vi "Config - Read.vi"(8 "error in (no error)":errorcluster, 11 "Filepath":path) -> (0 "error out":errorcluster, 3 "Config Array":T1 {"Balance" format="%9.2g"})   [LabVIEW 2017]
doc: "Provides READ all data from external config DB."
uses:
  Controls/Config Array.ctl
  Controls/Config Data.ctl
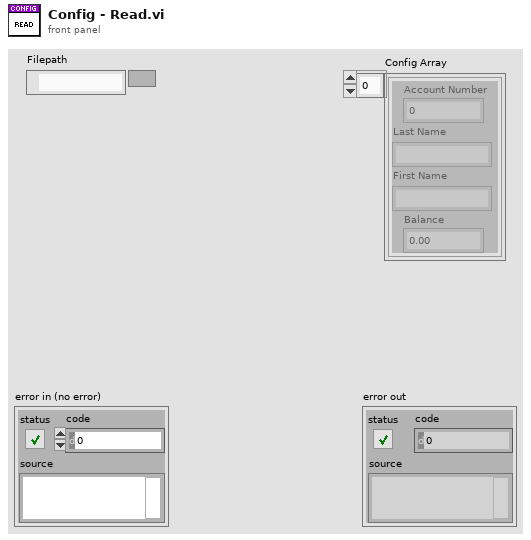
[diagram p1: front panel]
types:
  T1 = typedef "Config Array.ctl" = T2[]
  T2 = typedef "Config Data.ctl" = cluster{"Account Number":u32, "Last Name":string, "First Name":string, "Balance":dbl}
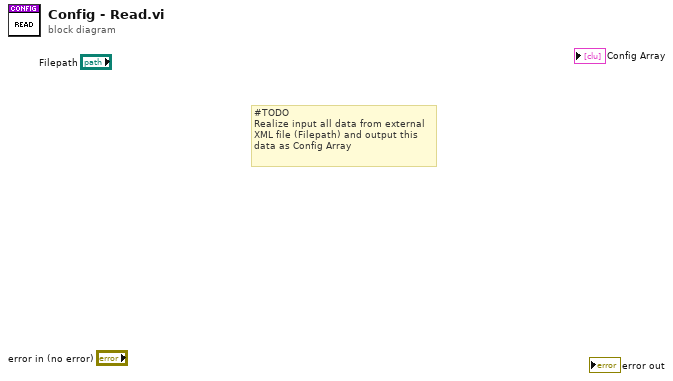
[diagram p0: block diagram]
diagram:
  # "#TODO\nRealize input all data from external\nXML file (Filepath) and output this\ndata as Config Array"
